vi "2CubeRoutineSelector.vi"(4 "Switch":bool, 5 "Scale":bool, 6 "Prior Routine File Name":string, 7 "GameData":string, 8 "RR":dbl, 9 "RL":dbl, 10 "LR":dbl, 11 "LL":dbl) -> (3 "File Path":string)   [LabVIEW 2017]
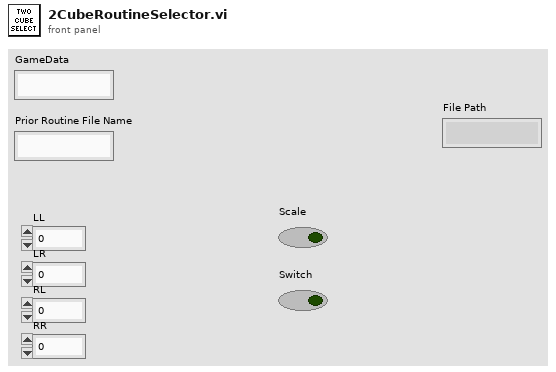
[diagram p1: front panel]
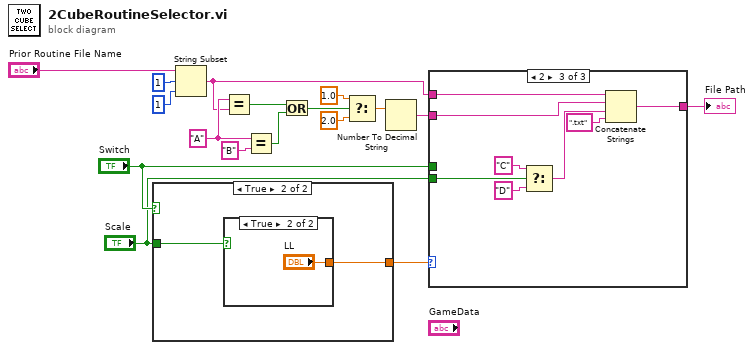
[diagram p0: block diagram]
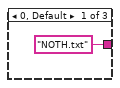
[diagram p2: hidden frame]
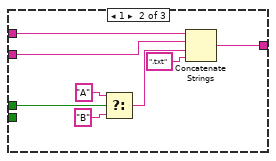
[diagram p3: hidden frame]
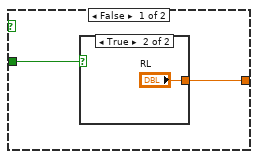
[diagram p4: hidden frame]
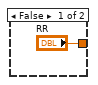
[diagram p5: hidden frame]
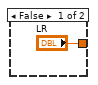
[diagram p6: hidden frame]
diagram:
  w11 = "A" ("x")
  n1 = case shown="True" "Switch" {
    tunnel: "Scale" -> [w19 w23]
    tunnel: [w18 w22] -> w6
    frame False {
      n2 = case shown="True" w19 {
        tunnel: ["RR" "RL"] -> w18
        frame False {
        }
        frame True {
        }
      }
    }
    frame True {
      n3 = case shown="True" w23 {
        tunnel: ["LR" "LL"] -> w22
        frame False {
        }
        frame True {
        }
      }
    }
  }
  n4 = String Subset(string="Prior Routine File Name", offset (0)=1, length (rest)=1 ("length (rest)")) -> (substring=w1:string)
  n5 = Equal?(x=w11, y=w1) -> (x = y?=w13:bool)
  n6 = Equal?(x=w11, y="B" ("x")) -> (x = y?=w14:bool)
  n7 = Or(x=w13, y=w14) -> (x .or. y?=w10:bool)
  n8 = Select(t=1.0, s=w10, f=2.0) -> (s? t:f=w7:dbl)
  n9 = Number To Decimal String(number=w7) -> (decimal integer string=w2:string)  [unwired: 1 in]
  n10 = case shown="2" w6 {
    tunnel: ["NOTH.txt" ("x") w27 w39] -> w3
    tunnel: "Switch" -> [_ w34 _]
    tunnel: "Scale" -> [_ _ w40]
    tunnel: w2 -> [_ w30 w36]
    tunnel: w1 -> [_ w29 w35]
    frame 0, Default {
    }
    frame 1 {
      n11 = Select(t="A" ("x"), s=w34, f="B" ("x")) -> (s? t:f=w31:string)
      n12 = Concatenate Strings(w29, w30, w31, ".txt" ("string")) -> (w27:string)
    }
    frame 2 {
      n13 = Select(t="C" ("x"), s=w40, f="D" ("x")) -> (s? t:f=w37:string)
      n14 = Concatenate Strings(w35, w36, w37, ".txt" ("string")) -> (w39:string)
    }
  }
  "File Path" <- w3
